vi "sub_find-pts.vi"() -> ()   [LabVIEW 2019]
uses:
  Ctrl/waypoint_buf.ctl
  Ctrl/points.ctl
  Ctrl/cmd_common.ctl
panel:
  out "waypoint analysis format":T1
  in  "wpt scan":bool
  out "part wpt":T2(graph)=[{"in circle waypts"=[{"x"=175263.821, "y"=530281.169}, {"x"=175263.854, "y"=530281.16}, {"x"=175263.883, "y"=530281.152}, {"x"=175263.908, "y"=530281.145}, {"x"=175263.932, "y"=530281.139}, {"x"=175263.96, "y"=530281.132}, {"x"=175263.991, "y"=530281.124}, {"x"=175264.027, "y"=530281.115}, {"x"=175264.063, "y"=530281.106}, {"x"=175264.096, "y"=530281.097}, {"x"=175264.127, "y"=530281.089}, {"x"=175264.155, "y"=530281.083}, {"x"=175264.182, "y"=530281.076}, {"x"=175264.209, "y"=530281.07}, {"x"=175264.235, "y"=530281.064}, {"x"=175264.263, "y"=530281.058}, {"x"=175264.291, "y"=530281.052}, {"x"=175264.319, "y"=530281.046}, {"x"=175264.346, "y"=530281.04}, {"x"=175264.375, "y"=530281.035}, {"x"=175264.407, "y"=530281.028}, {"x"=175264.443, "y"=530281.02}, {"x"=175264.479, "y"=530281.012}, {"x"=175264.516, "y"=530281.004}, {"x"=175264.552, "y"=530280.996}, {"x"=175264.586, "y"=530280.989}, {"x"=175264.617, "y"=530280.981}, {"x"=175264.645, "y"=530280.975}, {"x"=175264.67, "y"=530280.969}, {"x"=175264.696, "y"=530280.963}, {"x"=175264.721, "y"=530280.958}, {"x"=175264.746, "y"=530280.951}, {"x"=175264.772, "y"=530280.945}, {"x"=175264.8, "y"=530280.938}, {"x"=175264.83, "y"=530280.931}, {"x"=175264.86, "y"=530280.924}, {"x"=175264.893, "y"=530280.916}, {"x"=175264.926, "y"=530280.908}, {"x"=175264.961, "y"=530280.9}, {"x"=175264.996, "y"=530280.892}, {"x"=175265.03, "y"=530280.884}, {"x"=175265.064, "y"=530280.876}, {"x"=175265.097, "y"=530280.869}, {"x"=175265.129, "y"=530280.861}, {"x"=175265.16, "y"=530280.855}, {"x"=175265.189, "y"=530280.848}, {"x"=175265.217, "y"=530280.842}, {"x"=175265.245, "y"=530280.835}, {"x"=175265.274, "y"=530280.828}, {"x"=175265.304, "y"=530280.821}, {"x"=175265.336, "y"=530280.813}, {"x"=175265.37, "y"=530280.805}, {"x"=175265.406, "y"=530280.797}, {"x"=175265.441, "y"=530280.788}, {"x"=175265.477, "y"=530280.778}, {"x"=175265.513, "y"=530280.769}, {"x"=175265.547, "y"=530280.761}, {"x"=175265.579, "y"=530280.753}, {"x"=175265.61, "y"=530280.745}, {"x"=175265.639, "y"=530280.738}, {"x"=175265.667, "y"=530280.731}, {"x"=175265.695, "y"=530280.724}, {"x"=175265.722, "y"=530280.718}, {"x"=175265.752, "y"=530280.711}, {"x"=175265.784, "y"=530280.704}, {"x"=175265.818, "y"=530280.696}, {"x"=175265.854, "y"=530280.687}, {"x"=175265.891, "y"=530280.678}, {"x"=175265.928, "y"=530280.67}, {"x"=175265.964, "y"=530280.662}, {"x"=175266.0, "y"=530280.653}, {"x"=175266.035, "y"=530280.645}, {"x"=175266.068, "y"=530280.637}, {"x"=175266.099, "y"=530280.629}, {"x"=175266.129, "y"=530280.621}, {"x"=175266.159, "y"=530280.614}, {"x"=175266.19, "y"=530280.607}, {"x"=175266.221, "y"=530280.6}, {"x"=175266.254, "y"=530280.592}, {"x"=175266.289, "y"=530280.584}, {"x"=175266.324, "y"=530280.575}, {"x"=175266.36, "y"=530280.567}, {"x"=175266.397, "y"=530280.559}, {"x"=175266.432, "y"=530280.55}, {"x"=175266.467, "y"=530280.542}, {"x"=175266.501, "y"=530280.534}, {"x"=175266.533, "y"=530280.526}, {"x"=175266.565, "y"=530280.518}, {"x"=175266.596, "y"=530280.51}, {"x"=175266.627, "y"=530280.502}, {"x"=175266.66, "y"=530280.495}, {"x"=175266.694, "y"=530280.487}, {"x"=175266.729, "y"=530280.478}, {"x"=175266.765, "y"=530280.469}, {"x"=175266.801, "y"=530280.46}, {"x"=175266.837, "y"=530280.451}, {"x"=175266.873, "y"=530280.442}, {"x"=175266.909, "y"=530280.433}, {"x"=175266.944, "y"=530280.424}, {"x"=175266.979, "y"=530280.416}, {"x"=175267.013, "y"=530280.407}, {"x"=175267.048, "y"=530280.398}, {"x"=175267.083, "y"=530280.389}, {"x"=175267.12, "y"=530280.38}, {"x"=175267.157, "y"=530280.371}, {"x"=175267.194, "y"=530280.362}, {"x"=175267.233, "y"=530280.352}, {"x"=175267.271, "y"=530280.342}, {"x"=175267.308, "y"=530280.333}, {"x"=175267.344, "y"=530280.323}, {"x"=175267.38, "y"=530280.314}, {"x"=175267.416, "y"=530280.305}, {"x"=175267.451, "y"=530280.296}, {"x"=175267.488, "y"=530280.287}, {"x"=175267.526, "y"=530280.278}, {"x"=175267.565, "y"=530280.268}, {"x"=175267.604, "y"=530280.258}, {"x"=175267.645, "y"=530280.247}, {"x"=175267.686, "y"=530280.236}, {"x"=175267.726, "y"=530280.227}, {"x"=175267.766, "y"=530280.217}, {"x"=175267.803, "y"=530280.208}, {"x"=175267.84, "y"=530280.199}, {"x"=175267.876, "y"=530280.19}, {"x"=175267.91, "y"=530280.181}, {"x"=175267.945, "y"=530280.172}, {"x"=175267.979, "y"=530280.163}, {"x"=175268.012, "y"=530280.154}, {"x"=175268.044, "y"=530280.146}, {"x"=175268.077, "y"=530280.138}, {"x"=175268.113, "y"=530280.129}, {"x"=175268.151, "y"=530280.12}, {"x"=175268.189, "y"=530280.111}, {"x"=175268.226, "y"=530280.102}, {"x"=175268.262, "y"=530280.093}, {"x"=175268.294, "y"=530280.085}, {"x"=175268.325, "y"=530280.078}, {"x"=175268.358, "y"=530280.071}, {"x"=175268.394, "y"=530280.062}, {"x"=175268.432, "y"=530280.053}, {"x"=175268.47, "y"=530280.044}, {"x"=175268.508, "y"=530280.035}, {"x"=175268.545, "y"=530280.026}, {"x"=175268.578, "y"=530280.018}, {"x"=175268.607, "y"=530280.01}, {"x"=175268.635, "y"=530280.004}, {"x"=175268.666, "y"=530279.998}, {"x"=175268.7, "y"=530279.99}, {"x"=175268.737, "y"=530279.981}, {"x"=175268.775, "y"=530279.972}, {"x"=175268.814, "y"=530279.963}, {"x"=175268.853, "y"=530279.954}, {"x"=175268.892, "y"=530279.945}, {"x"=175268.926, "y"=530279.937}, {"x"=175268.956, "y"=530279.929}, {"x"=175268.984, "y"=530279.922}, {"x"=175269.015, "y"=530279.917}, {"x"=175269.049, "y"=530279.91}, {"x"=175269.084, "y"=530279.901}, {"x"=175269.121, "y"=530279.892}, {"x"=175269.158, "y"=530279.884}, {"x"=175269.194, "y"=530279.877}, {"x"=175269.225, "y"=530279.869}, {"x"=175269.253, "y"=530279.862}, {"x"=175269.282, "y"=530279.856}, {"x"=175269.315, "y"=530279.85}, {"x"=175269.352, "y"=530279.842}, {"x"=175269.393, "y"=530279.833}, {"x"=175269.434, "y"=530279.825}, {"x"=175269.474, "y"=530279.816}, {"x"=175269.512, "y"=530279.808}, {"x"=175269.544, "y"=530279.802}, {"x"=175269.571, "y"=530279.796}, {"x"=175269.598, "y"=530279.79}, {"x"=175269.63, "y"=530279.784}, {"x"=175269.666, "y"=530279.778}, {"x"=175269.705, "y"=530279.769}, {"x"=175269.745, "y"=530279.76}, {"x"=175269.787, "y"=530279.752}, {"x"=175269.827, "y"=530279.744}, {"x"=175269.866, "y"=530279.736}, {"x"=175269.902, "y"=530279.728}, {"x"=175269.937, "y"=530279.721}, {"x"=175269.969, "y"=530279.715}, {"x"=175270.0, "y"=530279.708}, {"x"=175270.029, "y"=530279.701}, {"x"=175270.057, "y"=530279.696}, {"x"=175270.086, "y"=530279.691}, {"x"=175270.114, "y"=530279.685}, {"x"=175270.144, "y"=530279.678}, {"x"=175270.177, "y"=530279.672}, {"x"=175270.211, "y"=530279.665}, {"x"=175270.248, "y"=530279.657}, {"x"=175270.285, "y"=530279.65}, {"x"=175270.322, "y"=530279.643}, {"x"=175270.36, "y"=530279.635}, {"x"=175270.396, "y"=530279.627}, {"x"=175270.432, "y"=530279.619}, {"x"=175270.467, "y"=530279.612}, {"x"=175270.5, "y"=530279.605}, {"x"=175270.533, "y"=530279.598}, {"x"=175270.564, "y"=530279.591}, {"x"=175270.596, "y"=530279.584}, {"x"=175270.628, "y"=530279.578}, {"x"=175270.66, "y"=530279.571}, {"x"=175270.694, "y"=530279.564}, {"x"=175270.728, "y"=530279.557}, {"x"=175270.762, "y"=530279.549}, {"x"=175270.796, "y"=530279.542}, {"x"=175270.83, "y"=530279.535}, {"x"=175270.864, "y"=530279.527}, {"x"=175270.899, "y"=530279.52}, {"x"=175270.934, "y"=530279.513}, {"x"=175270.969, "y"=530279.505}, {"x"=175271.003, "y"=530279.498}, {"x"=175271.037, "y"=530279.49}, {"x"=175271.072, "y"=530279.483}, {"x"=175271.107, "y"=530279.475}, {"x"=175271.142, "y"=530279.468}, {"x"=175271.178, "y"=530279.46}, {"x"=175271.213, "y"=530279.452}, {"x"=175271.248, "y"=530279.444}, {"x"=175271.282, "y"=530279.437}, {"x"=175271.316, "y"=530279.429}, {"x"=175271.351, "y"=530279.421}, {"x"=175271.385, "y"=530279.413}, {"x"=175271.421, "y"=530279.405}, {"x"=175271.456, "y"=530279.397}, {"x"=175271.493, "y"=530279.389}, {"x"=175271.53, "y"=530279.381}, {"x"=175271.567, "y"=530279.373}, {"x"=175271.604, "y"=530279.364}, {"x"=175271.64, "y"=530279.356}, {"x"=175271.674, "y"=530279.348}, {"x"=175271.708, "y"=530279.34}, {"x"=175271.74, "y"=530279.333}, {"x"=175271.771, "y"=530279.325}, {"x"=175271.803, "y"=530279.318}, {"x"=175271.834, "y"=530279.311}, {"x"=175271.867, "y"=530279.303}, {"x"=175271.902, "y"=530279.295}, {"x"=175271.937, "y"=530279.287}, {"x"=175271.974, "y"=530279.278}, {"x"=175272.011, "y"=530279.269}, {"x"=175272.047, "y"=530279.261}, {"x"=175272.08, "y"=530279.254}, {"x"=175272.112, "y"=530279.247}, {"x"=175272.146, "y"=530279.24}, {"x"=175272.181, "y"=530279.233}, {"x"=175272.216, "y"=530279.225}, {"x"=175272.251, "y"=530279.217}, {"x"=175272.286, "y"=530279.21}, {"x"=175272.32, "y"=530279.203}, {"x"=175272.351, "y"=530279.196}, {"x"=175272.381, "y"=530279.19}, {"x"=175272.411, "y"=530279.184}, {"x"=175272.443, "y"=530279.177}, {"x"=175272.479, "y"=530279.169}, {"x"=175272.517, "y"=530279.162}, {"x"=175272.555, "y"=530279.153}, {"x"=175272.592, "y"=530279.145}, {"x"=175272.628, "y"=530279.138}, {"x"=175272.661, "y"=530279.131}, {"x"=175272.692, "y"=530279.124}, {"x"=175272.719, "y"=530279.118}, {"x"=175272.742, "y"=530279.113}, {"x"=175272.764, "y"=530279.109}, {"x"=175272.787, "y"=530279.105}, {"x"=175272.815, "y"=530279.1}, {"x"=175272.846, "y"=530279.094}, {"x"=175272.88, "y"=530279.087}, {"x"=175272.915, "y"=530279.08}, {"x"=175272.95, "y"=530279.074}, {"x"=175272.984, "y"=530279.068}, {"x"=175273.017, "y"=530279.061}, {"x"=175273.049, "y"=530279.055}, {"x"=175273.08, "y"=530279.049}, {"x"=175273.111, "y"=530279.042}, {"x"=175273.141, "y"=530279.036}, {"x"=175273.172, "y"=530279.029}, {"x"=175273.202, "y"=530279.023}, {"x"=175273.234, "y"=530279.017}, {"x"=175273.266, "y"=530279.011}, {"x"=175273.299, "y"=530279.005}, {"x"=175273.333, "y"=530278.997}, {"x"=175273.367, "y"=530278.991}, {"x"=175273.401, "y"=530278.985}, {"x"=175273.435, "y"=530278.978}, {"x"=175273.467, "y"=530278.971}, {"x"=175273.498, "y"=530278.964}, {"x"=175273.529, "y"=530278.957}, {"x"=175273.529, "y"=530278.957}, {"x"=175273.498, "y"=530278.964}, {"x"=175273.467, "y"=530278.971}, {"x"=175273.435, "y"=530278.978}, {"x"=175273.401, "y"=530278.985}, {"x"=175273.367, "y"=530278.991}, {"x"=175273.333, "y"=530278.997}, {"x"=175273.299, "y"=530279.005}, {"x"=175273.266, "y"=530279.011}, {"x"=175273.234, "y"=530279.017}, {"x"=175273.202, "y"=530279.023}, {"x"=175273.172, "y"=530279.029}, {"x"=175273.141, "y"=530279.036}, {"x"=175273.111, "y"=530279.042}, {"x"=175273.08, "y"=530279.049}, {"x"=175273.049, "y"=530279.055}, {"x"=175273.017, "y"=530279.061}, {"x"=175272.984, "y"=530279.068}, {"x"=175272.95, "y"=530279.074}, {"x"=175272.915, "y"=530279.08}, {"x"=175272.88, "y"=530279.087}, {"x"=175272.846, "y"=530279.094}, {"x"=175272.815, "y"=530279.1}, {"x"=175272.787, "y"=530279.105}, {"x"=175272.764, "y"=530279.109}, {"x"=175272.742, "y"=530279.113}, {"x"=175272.719, "y"=530279.118}, {"x"=175272.692, "y"=530279.124}, {"x"=175272.661, "y"=530279.131}, {"x"=175272.628, "y"=530279.138}, {"x"=175272.592, "y"=530279.145}, {"x"=175272.555, "y"=530279.153}, {"x"=175272.517, "y"=530279.162}, {"x"=175272.479, "y"=530279.169}, {"x"=175272.443, "y"=530279.177}, {"x"=175272.411, "y"=530279.184}, {"x"=175272.381, "y"=530279.19}, {"x"=175272.351, "y"=530279.196}, {"x"=175272.32, "y"=530279.203}, {"x"=175272.286, "y"=530279.21}, {"x"=175272.251, "y"=530279.217}, {"x"=175272.216, "y"=530279.225}, {"x"=175272.181, "y"=530279.233}, {"x"=175272.146, "y"=530279.24}, {"x"=175272.112, "y"=530279.247}, {"x"=175272.08, "y"=530279.254}, {"x"=175272.047, "y"=530279.261}, {"x"=175272.011, "y"=530279.269}, {"x"=175271.974, "y"=530279.278}, {"x"=175271.937, "y"=530279.287}, {"x"=175271.902, "y"=530279.295}, {"x"=175271.867, "y"=530279.303}, {"x"=175271.834, "y"=530279.311}, {"x"=175271.803, "y"=530279.318}, {"x"=175271.771, "y"=530279.325}, {"x"=175271.74, "y"=530279.333}, {"x"=175271.708, "y"=530279.34}, {"x"=175271.674, "y"=530279.348}, {"x"=175271.64, "y"=530279.356}, {"x"=175271.604, "y"=530279.364}, {"x"=175271.567, "y"=530279.373}, {"x"=175271.53, "y"=530279.381}, {"x"=175271.493, "y"=530279.389}, {"x"=175271.456, "y"=530279.397}, {"x"=175271.421, "y"=530279.405}, {"x"=175271.385, "y"=530279.413}, {"x"=175271.351, "y"=530279.421}, {"x"=175271.316, "y"=530279.429}, {"x"=175271.282, "y"=530279.437}, {"x"=175271.248, "y"=530279.444}, {"x"=175271.213, "y"=530279.452}, {"x"=175271.178, "y"=530279.46}, {"x"=175271.142, "y"=530279.468}, {"x"=175271.107, "y"=530279.475}, {"x"=175271.072, "y"=530279.483}, {"x"=175271.037, "y"=530279.49}, {"x"=175271.003, "y"=530279.498}, {"x"=175270.969, "y"=530279.505}, {"x"=175270.934, "y"=530279.513}, {"x"=175270.899, "y"=530279.52}, {"x"=175270.864, "y"=530279.527}, {"x"=175270.83, "y"=530279.535}, {"x"=175270.796, "y"=530279.542}, {"x"=175270.762, "y"=530279.549}, {"x"=175270.728, "y"=530279.557}, {"x"=175270.694, "y"=530279.564}, {"x"=175270.66, "y"=530279.571}, {"x"=175270.628, "y"=530279.578}, {"x"=175270.596, "y"=530279.584}, {"x"=175270.564, "y"=530279.591}, {"x"=175270.533, "y"=530279.598}, {"x"=175270.5, "y"=530279.605}, {"x"=175270.467, "y"=530279.612}, {"x"=175270.432, "y"=530279.619}, {"x"=175270.396, "y"=530279.627}, {"x"=175270.36, "y"=530279.635}, {"x"=175270.322, "y"=530279.643}, {"x"=175270.285, "y"=530279.65}, {"x"=175270.248, "y"=530279.657}, {"x"=175270.211, "y"=530279.665}, {"x"=175270.177, "y"=530279.672}, {"x"=175270.144, "y"=530279.678}, {"x"=175270.114, "y"=530279.685}, {"x"=175270.086, "y"=530279.691}, {"x"=175270.057, "y"=530279.696}, {"x"=175270.029, "y"=530279.701}, {"x"=175270.0, "y"=530279.708}, {"x"=175269.969, "y"=530279.715}, {"x"=175269.937, "y"=530279.721}, {"x"=175269.902, "y"=530279.728}, {"x"=175269.866, "y"=530279.736}, {"x"=175269.827, "y"=530279.744}, {"x"=175269.787, "y"=530279.752}, {"x"=175269.745, "y"=530279.76}, {"x"=175269.705, "y"=530279.769}, {"x"=175269.666, "y"=530279.778}, {"x"=175269.63, "y"=530279.784}, {"x"=175269.598, "y"=530279.79}, {"x"=175269.571, "y"=530279.796}, {"x"=175269.544, "y"=530279.802}, {"x"=175269.512, "y"=530279.808}, {"x"=175269.474, "y"=530279.816}, {"x"=175269.434, "y"=530279.825}, {"x"=175269.393, "y"=530279.833}, {"x"=175269.352, "y"=530279.842}, {"x"=175269.315, "y"=530279.85}, {"x"=175269.282, "y"=530279.856}, {"x"=175269.253, "y"=530279.862}, {"x"=175269.225, "y"=530279.869}, {"x"=175269.194, "y"=530279.877}, {"x"=175269.158, "y"=530279.884}, {"x"=175269.121, "y"=530279.892}, {"x"=175269.084, "y"=530279.901}, {"x"=175269.049, "y"=530279.91}, {"x"=175269.015, "y"=530279.917}, {"x"=175268.984, "y"=530279.922}, {"x"=175268.956, "y"=530279.929}, {"x"=175268.926, "y"=530279.937}, {"x"=175268.892, "y"=530279.945}, {"x"=175268.853, "y"=530279.954}, {"x"=175268.814, "y"=530279.963}, {"x"=175268.775, "y"=530279.972}, {"x"=175268.737, "y"=530279.981}, {"x"=175268.7, "y"=530279.99}, {"x"=175268.666, "y"=530279.998}, {"x"=175268.635, "y"=530280.004}, {"x"=175268.607, "y"=530280.01}, {"x"=175268.578, "y"=530280.018}, {"x"=175268.545, "y"=530280.026}, {"x"=175268.508, "y"=530280.035}, {"x"=175268.47, "y"=530280.044}, {"x"=175268.432, "y"=530280.053}, {"x"=175268.394, "y"=530280.062}, {"x"=175268.358, "y"=530280.071}, {"x"=175268.325, "y"=530280.078}, {"x"=175268.294, "y"=530280.085}, {"x"=175268.262, "y"=530280.093}, {"x"=175268.226, "y"=530280.102}, {"x"=175268.189, "y"=530280.111}, {"x"=175268.151, "y"=530280.12}, {"x"=175268.113, "y"=530280.129}, {"x"=175268.077, "y"=530280.138}, {"x"=175268.044, "y"=530280.146}, {"x"=175268.012, "y"=530280.154}, {"x"=175267.979, "y"=530280.163}, {"x"=175267.945, "y"=530280.172}, {"x"=175267.91, "y"=530280.181}, {"x"=175267.876, "y"=530280.19}, {"x"=175267.84, "y"=530280.199}, {"x"=175267.803, "y"=530280.208}, {"x"=175267.766, "y"=530280.217}, {"x"=175267.726, "y"=530280.227}, {"x"=175267.686, "y"=530280.236}, {"x"=175267.645, "y"=530280.247}, {"x"=175267.604, "y"=530280.258}, {"x"=175267.565, "y"=530280.268}, {"x"=175267.526, "y"=530280.278}, {"x"=175267.488, "y"=530280.287}, {"x"=175267.451, "y"=530280.296}, {"x"=175267.416, "y"=530280.305}, {"x"=175267.38, "y"=530280.314}, {"x"=175267.344, "y"=530280.323}, {"x"=175267.308, "y"=530280.333}, {"x"=175267.271, "y"=530280.342}, {"x"=175267.233, "y"=530280.352}, {"x"=175267.194, "y"=530280.362}, {"x"=175267.157, "y"=530280.371}, {"x"=175267.12, "y"=530280.38}, {"x"=175267.083, "y"=530280.389}, {"x"=175267.048, "y"=530280.398}, {"x"=175267.013, "y"=530280.407}, {"x"=175266.979, "y"=530280.416}, {"x"=175266.944, "y"=530280.424}, {"x"=175266.909, "y"=530280.433}, {"x"=175266.873, "y"=530280.442}, {"x"=175266.837, "y"=530280.451}, {"x"=175266.801, "y"=530280.46}, {"x"=175266.765, "y"=530280.469}, {"x"=175266.729, "y"=530280.478}, {"x"=175266.694, "y"=530280.487}, {"x"=175266.66, "y"=530280.495}, {"x"=175266.627, "y"=530280.502}, {"x"=175266.596, "y"=530280.51}, {"x"=175266.565, "y"=530280.518}, {"x"=175266.533, "y"=530280.526}, {"x"=175266.501, "y"=530280.534}, {"x"=175266.467, "y"=530280.542}, {"x"=175266.432, "y"=530280.55}, {"x"=175266.397, "y"=530280.559}, {"x"=175266.36, "y"=530280.567}, {"x"=175266.324, "y"=530280.575}, {"x"=175266.289, "y"=530280.584}, {"x"=175266.254, "y"=530280.592}, {"x"=175266.221, "y"=530280.6}, {"x"=175266.19, "y"=530280.607}, {"x"=175266.159, "y"=530280.614}, {"x"=175266.129, "y"=530280.621}, {"x"=175266.099, "y"=530280.629}, {"x"=175266.068, "y"=530280.637}, {"x"=175266.035, "y"=530280.645}, {"x"=175266.0, "y"=530280.653}, {"x"=175265.964, "y"=530280.662}, {"x"=175265.928, "y"=530280.67}, {"x"=175265.891, "y"=530280.678}, {"x"=175265.854, "y"=530280.687}, {"x"=175265.818, "y"=530280.696}, {"x"=175265.784, "y"=530280.704}, {"x"=175265.752, "y"=530280.711}, {"x"=175265.722, "y"=530280.718}, {"x"=175265.695, "y"=530280.724}, {"x"=175265.667, "y"=530280.731}, {"x"=175265.639, "y"=530280.738}, {"x"=175265.61, "y"=530280.745}, {"x"=175265.579, "y"=530280.753}, {"x"=175265.547, "y"=530280.761}, {"x"=175265.513, "y"=530280.769}, {"x"=175265.477, "y"=530280.778}, {"x"=175265.441, "y"=530280.788}, {"x"=175265.406, "y"=530280.797}, {"x"=175265.37, "y"=530280.805}, {"x"=175265.336, "y"=530280.813}, {"x"=175265.304, "y"=530280.821}, {"x"=175265.274, "y"=530280.828}, {"x"=175265.245, "y"=530280.835}, {"x"=175265.217, "y"=530280.842}, {"x"=175265.189, "y"=530280.848}, {"x"=175265.16, "y"=530280.855}, {"x"=175265.129, "y"=530280.861}, {"x"=175265.097, "y"=530280.869}, {"x"=175265.064, "y"=530280.876}, {"x"=175265.03, "y"=530280.884}, {"x"=175264.996, "y"=530280.892}, {"x"=175264.961, "y"=530280.9}, {"x"=175264.926, "y"=530280.908}, {"x"=175264.893, "y"=530280.916}, {"x"=175264.86, "y"=530280.924}, {"x"=175264.83, "y"=530280.931}, {"x"=175264.8, "y"=530280.938}, {"x"=175264.772, "y"=530280.945}, {"x"=175264.746, "y"=530280.951}, {"x"=175264.721, "y"=530280.958}, {"x"=175264.696, "y"=530280.963}, {"x"=175264.67, "y"=530280.969}, {"x"=175264.645, "y"=530280.975}, {"x"=175264.617, "y"=530280.981}, {"x"=175264.586, "y"=530280.989}, {"x"=175264.552, "y"=530280.996}, {"x"=175264.516, "y"=530281.004}, {"x"=175264.479, "y"=530281.012}, {"x"=175264.443, "y"=530281.02}, {"x"=175264.407, "y"=530281.028}, {"x"=175264.375, "y"=530281.035}, {"x"=175264.346, "y"=530281.04}, {"x"=175264.319, "y"=530281.046}, {"x"=175264.291, "y"=530281.052}, {"x"=175264.263, "y"=530281.058}, {"x"=175264.235, "y"=530281.064}, {"x"=175264.209, "y"=530281.07}, {"x"=175264.182, "y"=530281.076}, {"x"=175264.155, "y"=530281.083}, {"x"=175264.127, "y"=530281.089}, {"x"=175264.096, "y"=530281.097}, {"x"=175264.063, "y"=530281.106}, {"x"=175264.027, "y"=530281.115}, {"x"=175263.991, "y"=530281.124}, {"x"=175263.96, "y"=530281.132}, {"x"=175263.932, "y"=530281.139}, {"x"=175263.908, "y"=530281.145}, {"x"=175263.883, "y"=530281.152}, {"x"=175263.854, "y"=530281.16}, {"x"=175263.821, "y"=530281.169}]}, {"in circle waypts"=[{"x"=175263.821, "y"=530281.169}]}]
  out "XYwpt":cluster{cluster{dbl, dbl}[]}[](graph)
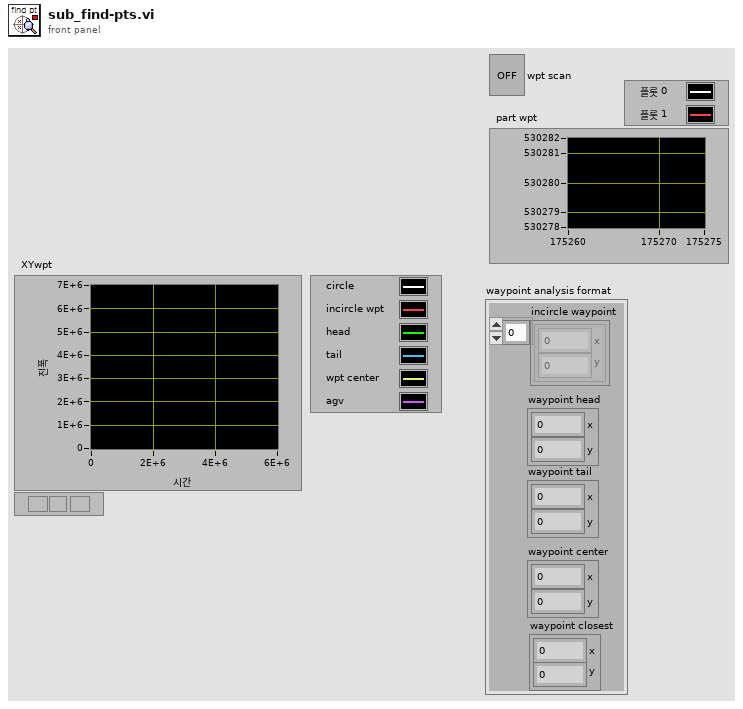
[diagram p1: front panel]
types:
  T1 = cluster{"incircle waypoint":cluster{"x":dbl, "y":dbl}[], "waypoint head":cluster{"x":dbl, "y":dbl}, "waypoint tail":cluster{"x":dbl, "y":dbl}, "waypoint center":cluster{"x":dbl, "y":dbl}, "waypoint closest":cluster{"x":dbl, "y":dbl}}
  T2 = cluster{"in circle waypts":cluster{"x":dbl, "y":dbl}[]}[]
  T3 = typedef "waypoint_buf.ctl" = enum16{"clear", "write", "read"}
  T4 = cluster{"lookahead pt n":dbl, "lookahead distance":dbl}
  T5 = cluster{"incircle waypoint":cluster{"x":dbl, "y":dbl}[]}
  T6 = cluster{"incircle waypoint":cluster{"x":dbl, "y":dbl}[]}[]
  T7 = cluster{"incircle waypoints":cluster{dbl, dbl}[]}
  T8 = typedef "cmd_common.ctl" = enum16{"read", "write"}
  T9 = typedef "points.ctl" = enum16{"read", "lookahead circle in", "lookahead in", "looktail in", "center in", "closest"}
  T10 = cluster{"lookahead":cluster{"x":dbl, "y":dbl}, "looktail":cluster{"x":dbl, "y":dbl}, "lookahead circle in":cluster{"x":dbl, "y":dbl}[], "center":cluster{"x":dbl, "y":dbl}, "wpt closest":cluster{"x":dbl, "y":dbl}}
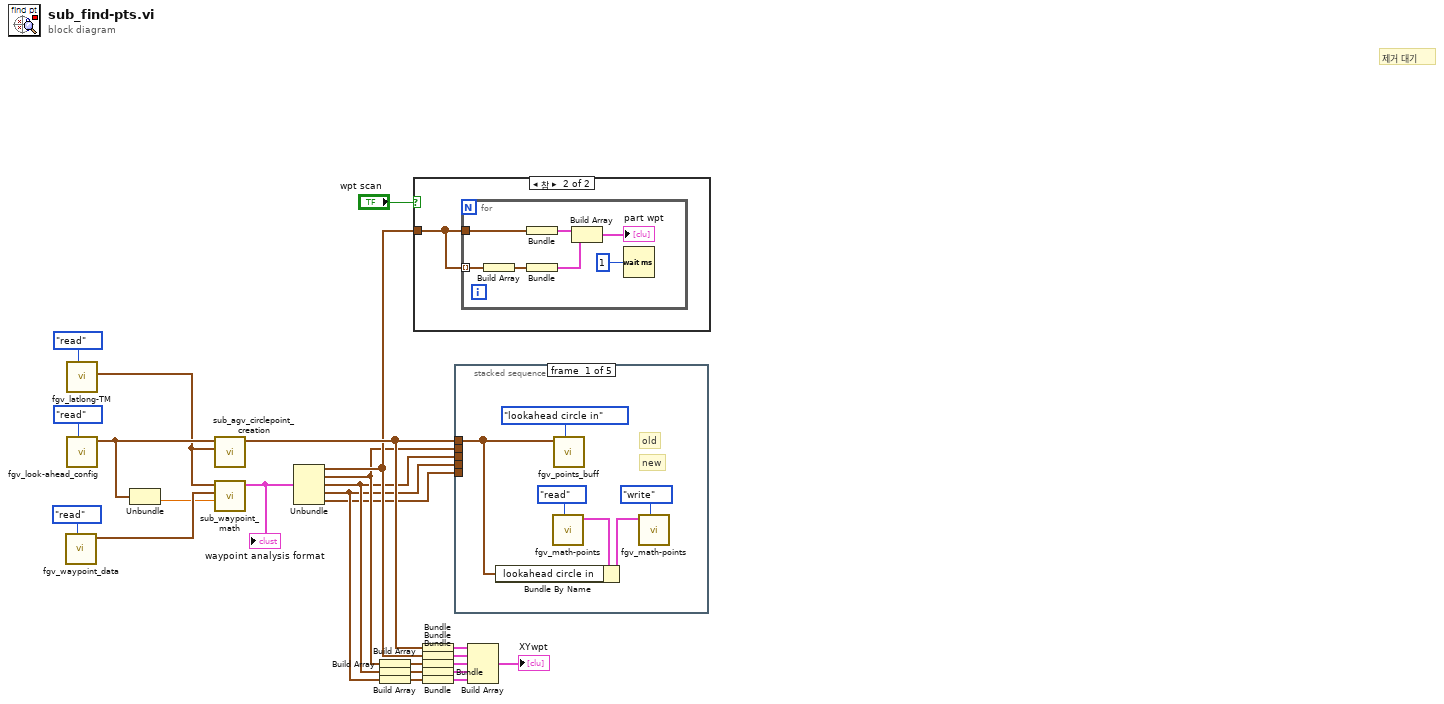
[diagram p0: block diagram]
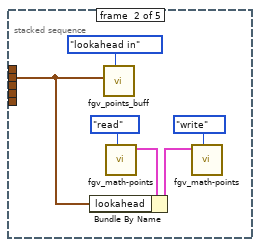
[diagram p2: hidden frame]
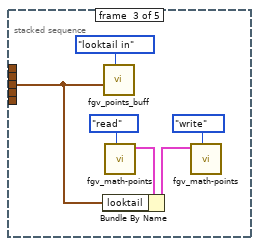
[diagram p3: hidden frame]
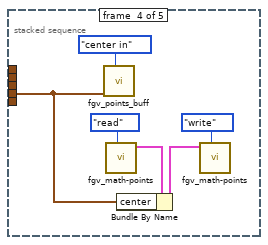
[diagram p4: hidden frame]
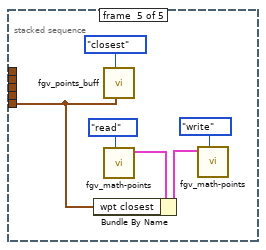
[diagram p5: hidden frame]
diagram:
  # "제거 대기"
  n1 = call "fgv_waypoint_data.vi"("cmd"=waypoint_buf."read") -> ("waypoint out"=w10:cluster{"x":dbl, "y":dbl}[])  [unwired: 8 in, 2 out]
  n2 = call "fgv_latlong-TM.vi"("cmd"=enum16{"write", "read"}."read") -> ("tm out"=w1:cluster{"YE":dbl, "XN":dbl})  [unwired: 9 in, 1 out]
  n3 = call "fgv_look-ahead_config.vi"("cmd"=enum16{"read", "write"}."read") -> ("lookahed cfg out"=w9:T4)  [unwired: 10 in]
  n4 = Unbundle(w9) -> ("lookahead distance"=w8:dbl)  [unwired: 1 out]
  n5 = call "sub_agv_circlepoint_creation.vi"("tm out"=w1, "lookahed cfg out"=w9) -> ("incircle waypoints"=w11:cluster{dbl, dbl}[])  [unwired: 9 in]
  n6 = call "sub_waypoint_math.vi"("lookahead distance"=w8, "waypoint out"=w10, "tm out"=w1) -> ("waypoint analysis format"=w7:T1)  [unwired: 8 in]
  "waypoint analysis format" <- w7
  n7 = Unbundle(w7) -> ("incircle waypoint"=w6:cluster{"x":dbl, "y":dbl}[], "waypoint head"=w5:cluster{"x":dbl, "y":dbl}, "waypoint tail"=w4:cluster{"x":dbl, "y":dbl}, "waypoint center"=w3:cluster{"x":dbl, "y":dbl}, "waypoint closest"=w2:cluster{"x":dbl, "y":dbl})
  n8 = Build Array(w5) -> (w18:cluster{"x":dbl, "y":dbl}[])
  n9 = Build Array(w4) -> (w19:cluster{"x":dbl, "y":dbl}[])
  n10 = Build Array(w3) -> (w13:cluster{"x":dbl, "y":dbl}[])
  n11 = case shown="참" "wpt scan" {
    tunnel: w6 -> [_ w25]
    frame False {
    }
    frame True {
      n12 = for {
        tunnel: w25 -> [w31] mode=indexing
        tunnel: w25 -> [w32]
        n13 = Build Array(w31) -> (w30:cluster{"x":dbl, "y":dbl}[])
        n14 = Bundle("incircle waypoint"=w32) -> (w28:T5)  [unwired: 1 in]
        n15 = Bundle(w30) -> (w29:cluster{cluster{"x":dbl, "y":dbl}[]})  [unwired: 1 in]
        n16 = Build Array(w28, w29) -> (→"part wpt":T6)
        n17 = Wait (ms)(milliseconds to wait=u32 1 ("dt")) -> ()  [unwired: 1 out]
      }
    }
  }
  n18 = Bundle("incircle waypoints"=w11) -> (w21:T7)  [unwired: 1 in]
  n19 = Bundle("incircle waypoint"=w6) -> (w20:T5)  [unwired: 1 in]
  n20 = Bundle(w18) -> (w17:cluster{cluster{"x":dbl, "y":dbl}[]})  [unwired: 1 in]
  n21 = Bundle(w19) -> (w16:cluster{cluster{"x":dbl, "y":dbl}[]})  [unwired: 1 in]
  n22 = Bundle(w13) -> (w14:cluster{cluster{"x":dbl, "y":dbl}[]})  [unwired: 1 in]
  n23 = stacked-sequence {
    tunnel: w11 -> [w33 _ _ _ _]
    tunnel: w5 -> [_ w39 _ _ _]
    tunnel: w3 -> [_ _ _ w51 _]
    tunnel: w4 -> [_ _ w45 _ _]
    tunnel: w2 -> [_ _ _ _ w58]
    frame #0 {
      # "new"
      # "old"
      n24 = call "fgv_math-points.vi"("cmd"=cmd_common."read") -> ("point-db out"=w35:T10)  [unwired: 10 in]
      n25 = Bundle By Name(cluster=w35, "lookahead circle in"=w33) -> (w34:T10)
      n26 = call "fgv_points_buff.vi"("cmd"=points."lookahead circle in", "lookahead circle in"=w33) -> ()  [unwired: 5 in, 5 out]
      n27 = call "fgv_math-points.vi"("cmd"=cmd_common."write", "point-db"=w34) -> ()  [unwired: 9 in, 1 out]
    }
    frame #1 {
      n28 = call "fgv_points_buff.vi"("cmd"=points."lookahead in", "lookahead in"=w39) -> ()  [unwired: 5 in, 5 out]
      n29 = call "fgv_math-points.vi"("cmd"=cmd_common."read") -> ("point-db out"=w41:T10)  [unwired: 10 in]
      n30 = Bundle By Name(cluster=w41, "lookahead"=w39) -> (w40:T10)
      n31 = call "fgv_math-points.vi"("cmd"=cmd_common."write", "point-db"=w40) -> ()  [unwired: 9 in, 1 out]
    }
    frame #2 {
      n32 = call "fgv_points_buff.vi"("cmd"=points."looktail in", "looktail in"=w45) -> ()  [unwired: 5 in, 5 out]
      n33 = call "fgv_math-points.vi"("cmd"=cmd_common."read") -> ("point-db out"=w47:T10)  [unwired: 10 in]
      n34 = Bundle By Name(cluster=w47, "looktail"=w45) -> (w46:T10)
      n35 = call "fgv_math-points.vi"("cmd"=cmd_common."write", "point-db"=w46) -> ()  [unwired: 9 in, 1 out]
    }
    frame #3 {
      n36 = call "fgv_points_buff.vi"("cmd"=points."center in", "center in"=w51) -> ()  [unwired: 5 in, 5 out]
      n37 = call "fgv_math-points.vi"("cmd"=cmd_common."read") -> ("point-db out"=w53:T10)  [unwired: 10 in]
      n38 = Bundle By Name(cluster=w53, "center"=w51) -> (w52:T10)
      n39 = call "fgv_math-points.vi"("cmd"=cmd_common."write", "point-db"=w52) -> ()  [unwired: 9 in, 1 out]
    }
    frame #4 {
      n40 = call "fgv_points_buff.vi"("closest in"=w58, "cmd"=points."closest") -> ()  [unwired: 5 in, 5 out]
      n41 = call "fgv_math-points.vi"("cmd"=cmd_common."read") -> ("point-db out"=w60:T10)  [unwired: 10 in]
      n42 = Bundle By Name(cluster=w60, "wpt closest"=w58) -> (w59:T10)
      n43 = call "fgv_math-points.vi"("cmd"=cmd_common."write", "point-db"=w59) -> ()  [unwired: 9 in, 1 out]
    }
  }
  n44 = Build Array(w21, w20, w17, w16, w14) -> (→"XYwpt":T6)
